vi "Obtain Receive Queue Reference.vi"(8 "Error In":errorcluster, 11 "Aircraft Index":u8) -> (0 "error out":errorcluster, 3 "Rx queue out":refnum<queue>)   [LabVIEW 2014]
uses:
  Aircraft Data Router/SubVI/Queue References/SubVI/Get Aircraft RX Queue String.vi
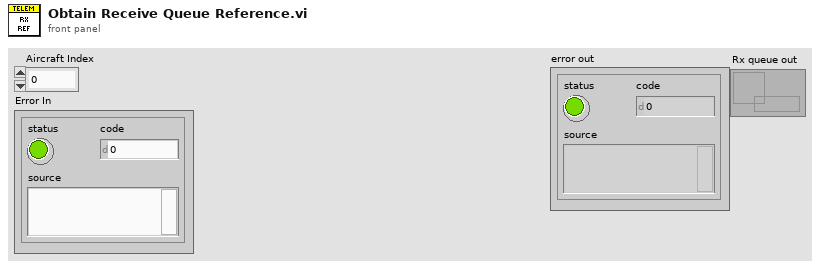
[diagram p1: front panel]
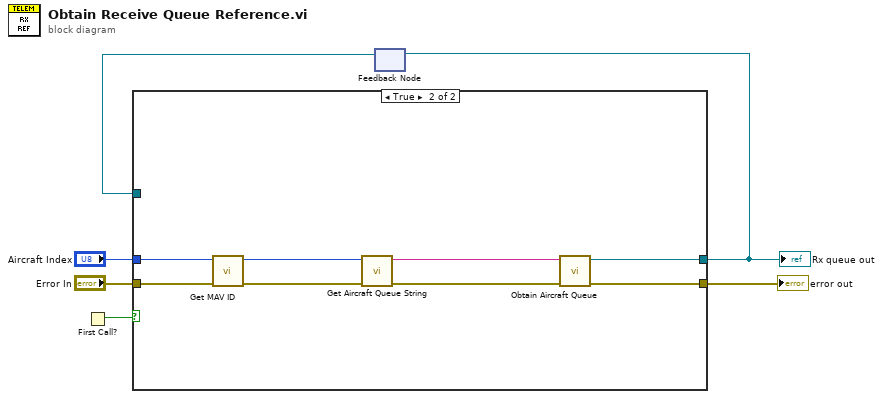
[diagram p0: block diagram]
diagram:
  n1 = First Call?() -> (First Call?: T/F=w4:bool)
  n2 = feedback #1() -> (w2:refnum<queue>)  [unwired: 1 in]
  n3 = case shown="True" w4 {
    tunnel: "Aircraft Index" -> [_ w14]
    tunnel: "Error In" -> [w8 w11]
    tunnel: [w8 w10] -> w1
    tunnel: [w7 w9] -> w3
    tunnel: w2 -> [w7 _]
    frame False {
    }
    frame True {
      n4 = call "Get MAV ID.vi"("Error In"=w11, "Aircraft Index"=w14) -> ("Error Out"=w13:errorcluster, "Aircraft ID"=w15:u8)  [unwired: 8 in]
      n5 = call-poly "Get Aircraft Queue String.vi"("Error In"=w13, "Aircraft ID"=w15) -> ("Error Out"=w12:errorcluster, "Aircraft Q Name"=w16:string)  [unwired: 8 in]
      n6 = call "Obtain Aircraft Queue.vi"("error in (no error)"=w12, "Queue Name"=w16) -> ("error out"=w10:errorcluster, "queue out"=w9:refnum<queue>)  [unwired: 8 in]
    }
  }
  "error out" <- w1
  "Rx queue out" <- w3
  n7 = feedback-in #1(w3) -> ()
